vi "Transmitter_Example.vi"() -> ()   [LabVIEW 2014]
uses:
  <instrlib>/niUSRP/niUSRP Write Tx Data (CDB).vi
panel:
  in  "upsampling number":i32=10
  out "Waveform Graph":cluster{"t0":dbl, "dt":dbl, "Y":dbl[]}(graph)
  in  "stop":bool
  in  "String":string="如果采用顺序流接收的方式：先从USRP缓存区获取数据，分局数据确定物理层分组，再将分组传给下面的解调模块。由于解码耗时较长，会拖累获取数据的速度，使得从USRP缓存区获取数据的速率低于采样率，从而引发缓冲区爆满的问题。\n那么将接收和解调使用并行运行的方式：一个线程获取缓存区数据，并根据信号强度抽取出一个物理层分组，将分组放到共享队列里面；另一个线程监听该队列，一旦获取一个分组，就进行解调和解码。这种方式可以有效地解决缓存区爆满的问题。\n我真是太TM机制了"
  out "USRP CoercedParamters":T1={"coerced IQ rate"=100000.0, "coerced carrier frequency"=100000.0, "coerced gain"=0.0} {"coerced gain" format="%#_6f"; "coerced carrier frequency" format="%#_6p"; "coerced IQ rate" format="%#_6p"}
  out "error out":errorcluster
  in  "error in (no error)":errorcluster
  in  "USRP ControledParameters":T2={"active antenna"="TX1", "gain"=30.0, "carrier frequency"=5800000000.0, "IQ rate"=2000000.0} {"IQ rate" format="%#_6p"; "carrier frequency" format="%#_6p"; "gain" format="%#_6f"}
  in  "device names":refnum<k15>="NI2900"
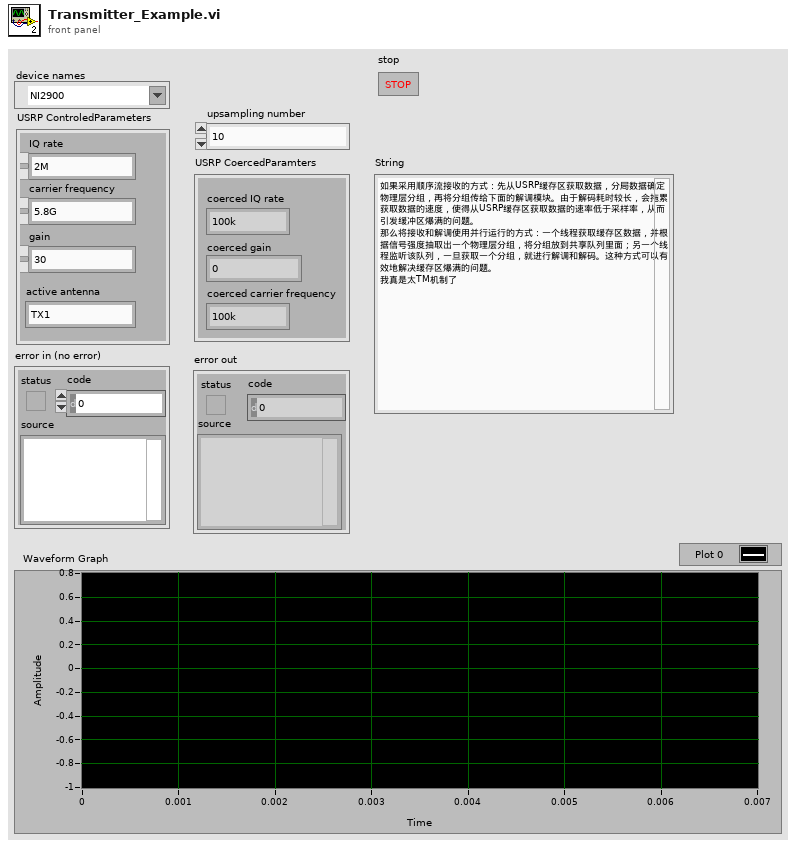
[diagram p1: front panel]
types:
  T1 = cluster{"coerced IQ rate":dbl, "coerced carrier frequency":dbl, "coerced gain":dbl}
  T2 = cluster{"active antenna":string, "gain":dbl, "carrier frequency":dbl, "IQ rate":dbl}
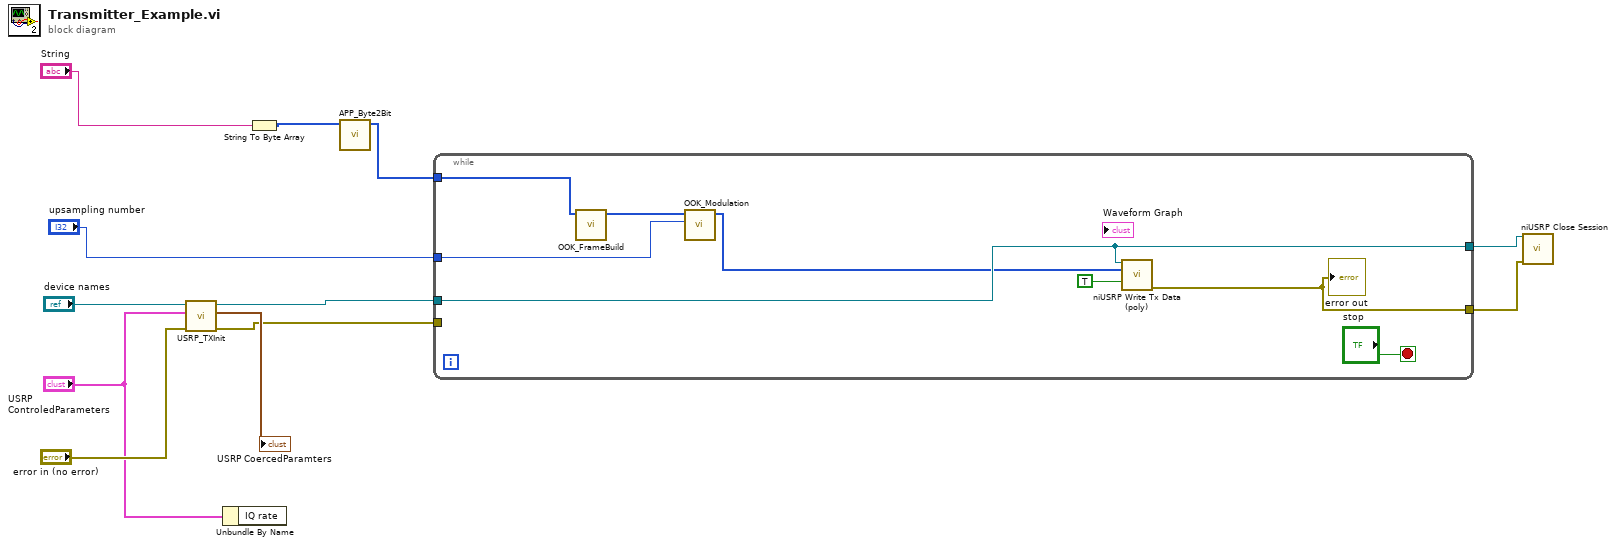
[diagram p0: block diagram]
diagram:
  n1 = call "USRP_TXInit.vi"("device names"="device names", "USRP ControledParameters"="USRP ControledParameters", "error in (no error)"="error in (no error)") -> ("session handle out"=w10:refnum<k15>, "USRP CoercedParamters"=→"USRP CoercedParamters":T1, "error out"=w7:errorcluster)  [unwired: 5 in]
  n2 = Unbundle By Name("USRP ControledParameters") -> ()  [unwired: 1 out]
  n3 = String To Byte Array(string="String") -> (unsigned byte array=w3:u8[])
  n4 = call "APP_Byte2Bit.vi"("input byte stream"=w3) -> ("output bit stream"=w4:i8[])  [unwired: 10 in]
  n5 = while {
    tunnel: w10 -> [w19]
    tunnel: w7 -> [_]
    tunnel: [w19] -> w6
    tunnel: [w18] -> w5
    tunnel: w4 -> [w17]
    tunnel: "upsampling number" -> [w15]
    stop <- "stop" stop-if-true
    n6 = call "OOK_FrameBuild.vi"("input bit stream"=w17) -> ("output bit stream"=w16:i8[])  [unwired: 10 in]
    n7 = call "OOK_Modulation.vi"("upsampling number"=w15, "input bit stream"=w16) -> ("output bit stream"=w13:i8[])  [unwired: 9 in]
    n8 = call-poly <instrlib>:"niUSRP Write Tx Data (poly).vi"("session handle"=w19, "data"=w13, "end of data?"=TRUE) -> ("error out"=w18:errorcluster)  [unwired: 11 in, 1 out]
    "error out" <- w18
  }
  n9 = call <instrlib>:"niUSRP Close Session.vi"("session handle"=w6, "error in (no error)"=w5) -> ()  [unwired: 13 in, 1 out]
